vi "Load and init CW laser.vi"(11 "path in":path=path "C:/SpinCore/SpinAPI/dll/spinapi64.dll") -> ()   [LabVIEW 2012]
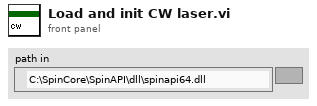
[diagram p1: front panel]
types:
  T1 = enum16{"Pulse Program", "Frequency Registers", "TX Phase Registers", "RX Phase Registers"}
  T2 = cluster{"Instruct Data":i32, "Op Code":i32, "Flags":bool[], "Comments":string, "Time (s)":dbl}[]
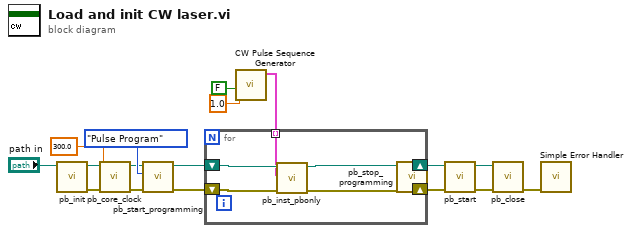
[diagram p0: block diagram]
diagram:
  n1 = call "pb_init.vi"("path in"="path in") -> ("error out"=w8:errorcluster, "path out"=w10:path)  [unwired: 3 in, 6 out]
  n2 = call "pb_core_clock.vi"("error in (no error)"=w8, "clock_freq (MHz)"=300.0, "path in"=w10) -> ("error out"=w7:errorcluster, "path out"=w9:path)  [unwired: 7 in]
  n3 = call "pb_start_programming.vi"("error in (no error)"=w7, "Device"=T1."Pulse Program", "path in"=w9) -> ("error out"=w4:errorcluster, "path out"=w5:path)  [unwired: 1 in, 6 out]
  n4 = call "CW Pulse Sequence Generator.vi"("Pulse MW"=FALSE, "Rate (Hz)"=1.0) -> ("Pulse Sequence Out"=w14:T2)  [unwired: 8 in]
  n5 = for {
    shift-right: [w22] -> w3
    shift-left: w5 -> [w24]
    shift-right: [w21] -> w2
    shift-left: w4 -> [w23]
    tunnel: w14 -> [w20] mode=indexing
    n6 = call "pb_inst_pbonly.vi"("error in (no error)"=w23, "PB Instruction"=w20, "path in"=w24) -> ("error out"=w21:errorcluster, "path out"=w22:path)  [unwired: 2 in, 5 out]
  }
  n7 = call "pb_stop_programming.vi"("error in (no error)"=w2, "path in"=w3) -> ("error out"=w17:errorcluster, "path out"=w15:path)  [unwired: 1 in, 7 out]
  n8 = call "pb_start.vi"("error in (no error)"=w17, "path in"=w15) -> ("error out"=w18:errorcluster, "path out"=w16:path)  [unwired: 1 in, 7 out]
  n9 = call "pb_close.vi"("error in (no error)"=w18, "path in"=w16) -> ("error out"=w19:errorcluster)  [unwired: 9 out]
  n10 = call <vilib>:"Simple Error Handler.vi"("error in (no error)"=w19) -> ()  [unwired: 1 in, 8 out]
